vi "save poc.vi"(8 "error in":errorcluster, 10 "path":string, 11 "power monitor queue in":refnum<queue>) -> (0 "error out":errorcluster)   [LabVIEW 2025, in "Automotive Vision.lvclass"]
uses:
  Automotive Vision.lvclass
  power.ctl
  Automotive Vision.lvclass/Automotive Vision.ctl
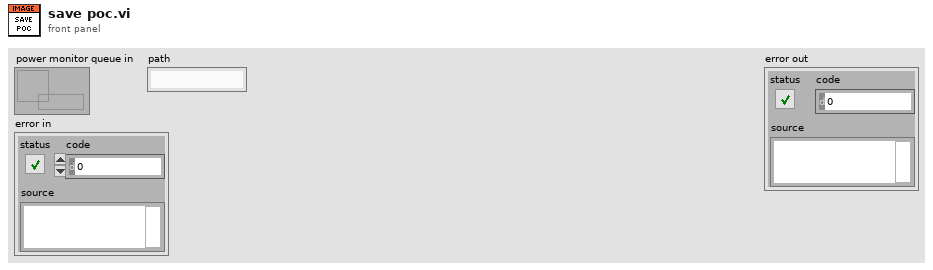
[diagram p1: front panel]
types:
  T1 = enum16{"open", "replace", "create", "open or create", "replace or create", "replace or create with confirmation"}
  T2 = typedef "Automotive Vision.lvclass/power.ctl" = cluster{"Voltage":dbl, "Current":dbl}
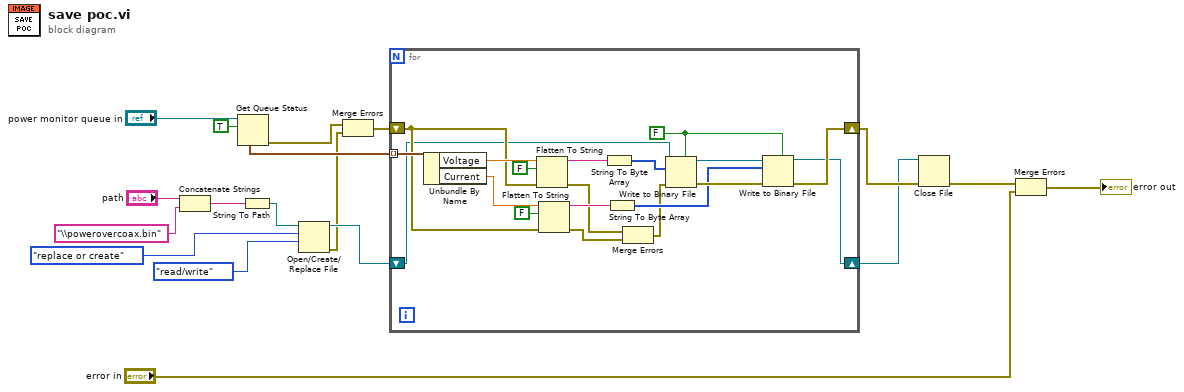
[diagram p0: block diagram]
diagram:
  n1 = Concatenate Strings("path", "\\powerovercoax.bin" ("element")) -> (w3:string)
  n2 = Get Queue Status(queue="power monitor queue in", return elements? (F)=TRUE) -> (error out=w11:errorcluster, elements=w14:T2[])  [unwired: 1 in, 6 out]
  n3 = String To Path(string=w3) -> (path=w2:path)
  n4 = Open/Create/Replace File(file path (use dialog)=w2, operation (0:open)=T1."replace or create", access (0:read/write)=enum16{"read/write", "read-only", "write-only"}."read/write") -> (refnum out=w13:refnum<file>, error out=w12:errorcluster)  [unwired: 3 in, 1 out]
  n5 = Merge Errors(w11, w12) -> (w10:errorcluster)
  n6 = for {
    tunnel: w14 -> [w37] mode=indexing
    shift-right: [w23] -> w7
    shift-left: w10 -> [w33]
    shift-right: [w19] -> w1
    shift-left: w13 -> [w28]
    w27 = FALSE ("prepend array or string size? (T)")
    n7 = Unbundle By Name(w37) -> ("Voltage"=w36:dbl, "Current"=w32:dbl)
    n8 = Flatten To String(anything=w36, prepend array or string size? (T)=FALSE, error in (no error)=w33) -> (data string=w31:string, error out=w21:errorcluster)  [unwired: 1 in, 1 out]
    n9 = Flatten To String(anything=w32, prepend array or string size? (T)=FALSE, error in (no error)=w33) -> (data string=w30:string, error out=w22:errorcluster)  [unwired: 1 in, 1 out]
    n10 = String To Byte Array(string=w31) -> (unsigned byte array=w29:u8[])
    n11 = String To Byte Array(string=w30) -> (unsigned byte array=w25:u8[])
    n12 = Merge Errors(w21, w22) -> (w20:errorcluster)
    n13 = Write to Binary File(file (use dialog)=w28, data=w29, error in=w20, 5:w27) -> (refnum out=w24:refnum<file>, error out=w26:errorcluster)  [unwired: 2 in, 1 out]
    n14 = Write to Binary File(file (use dialog)=w24, data=w25, error in=w26, 5:w27) -> (refnum out=w19:refnum<file>, error out=w23:errorcluster)  [unwired: 2 in, 1 out]
  }
  n15 = Close File(refnum=w1, error in=w7) -> (error out=w6:errorcluster)  [unwired: 1 out]
  n16 = Merge Errors(w6, "error in") -> (→"error out":errorcluster)
